vi "Set Configuration.vi"(8 "error in (no error)":errorcluster, 10 "Config name":string, 11 "Config in":refnum<class "Config.lvclass">) -> (0 "error out":errorcluster, 2 "All parameters":string[][](array[string]), 3 "Config out":refnum<class "Config.lvclass">)   [LabVIEW 2026, in "TALOS.lvlib" / "Classes.lvlib" / "Config.lvclass"]
doc: "This VI sets the current configuration to the one specified in input, if found among the available ones. If no value is provided, a \"default\" string is used.\nIt also returns the list of parameters with values for the specified configuration."
uses:
  Config.lvclass
  Config.lvclass/Config.ctl
  Ancestor/Ancestor/Ancestor.lvclass/Ancestor.ctl
  FGV/Error Memory/Get Error Description.vi
  Support VIs/Get PC name.vi
  Ancestor/Ancestor/Read ID.vi
  Support VIs/Get Class Name.vi
  <vilib>/Utility/error.llb/Clear Errors.vi
  FGV/Error Memory/Error Memory Core.vi
  <vilib>/AdvancedString/Delimited String to 1D String Array.vi
  <vilib>/AdvancedString/Delimited String to 1D String Array (string).vi
  Support VIs/Circus Root Path.vi
  FGV/Error Memory/Error Crt Lvl checker.vi
  FGV/Error Memory/Error Memory Core.vi/40c8088d-b597-4017-91af-faa98e00292e.vi
  FGV/Error Memory/Error Memory Core.vi/d4a3ab98-063c-4e44-b43d-fbdcfe6c2be2.vi
  Support VIs/Global Memory.vi
  <vilib>/Utility/LVClass/Get LV Class Name.vi
  Support VIs/Is in Packed Library.vi
  Support VIs/TALOS Root path.vi
  Support VIs/Read CSV worksheet.vi
  Support VIs/Global Constants.vi
  <vilib>/Utility/error.llb/General Error Handler.vi
  Ancestor/Ancestor/Ancestor.lvclass
  <vilib>/Comparison/Equal/Equal Functor/Equal Functor.lvclass
  TALOS.lvlib
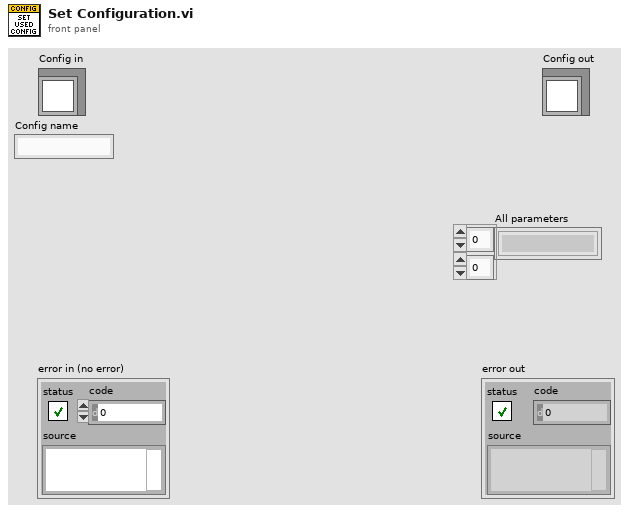
[diagram p1: front panel]
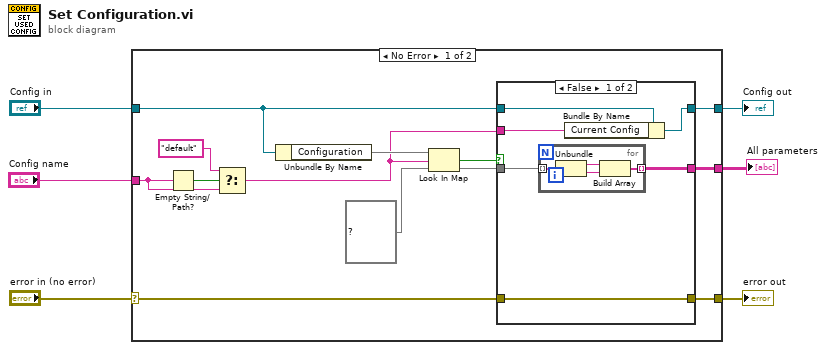
[diagram p0: block diagram]
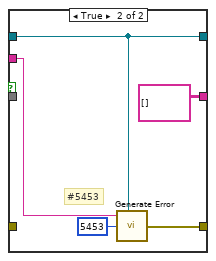
[diagram p2: hidden frame]
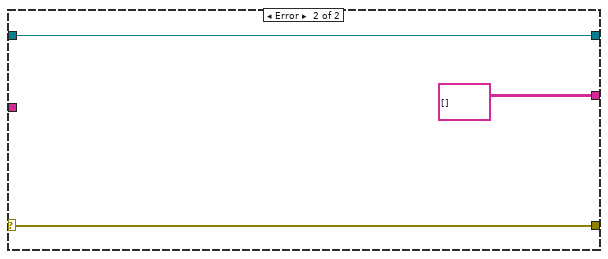
[diagram p3: hidden frame]
diagram:
  n1 = case shown="No Error" "error in (no error)" {
    selector: "error in (no error)" -> [w14 w37]
    tunnel: [w17 w37] -> w5
    tunnel: [w15 w36] -> w3
    tunnel: "Config in" -> [w16 w36]
    tunnel: "Config name" -> [w9 _]
    tunnel: [w12 string[][] [] ("Parameters")] -> w1
    frame No Error {
      n2 = Empty String/Path?(string/path=w9) -> (empty?=w11:bool)
      n3 = Select(t="default", s=w11, f=w9) -> (s? t:f=w10:string)
      n4 = Unbundle By Name(w16) -> ("Configuration"=w19:map{string, map{string, string}})
      n5 = Look In Map(map=w19, key=w10, default value=map{string, string} {}) -> (key not found?=w18:bool, value=w13:map{string, string})
      n6 = case shown="False" w18 {
        tunnel: [w25 w33] -> w17
        tunnel: w16 -> [w24 w31]
        tunnel: [w23 w31] -> w15
        tunnel: w14 -> [w25 _]
        tunnel: w10 -> [w22 w32]
        tunnel: w13 -> [w21 _]
        tunnel: [w20 string[][] []] -> w12
        frame False {
          n7 = for {
            tunnel: w21 -> [w29] mode=indexing
            tunnel: [w26] -> w20 mode=indexing
            n8 = Unbundle(w29) -> ("Key"=w28:string, "Value"=w27:string)
            n9 = Build Array(w28, w27) -> (w26:string[])
          }
          n10 = Bundle By Name(cluster=w24, "Current Config"=w22) -> (w23:refnum<class "Config.lvclass">)
        }
        frame True {
          # "#5453"
          n11 = call "Generate Error.vi"("Optional String"=w32, "Class"=w31, "Error Code"=5453) -> ("error out"=w33:errorcluster)  [unwired: 4 in]
        }
      }
    }
    frame Error {
    }
  }
  "error out" <- w5
  "Config out" <- w3
  "All parameters" <- w1
